vi "Untitled 2.vi"() -> ()   [LabVIEW 2020]
panel:
  in  "Numeric":i32
  out "XY Graph":cluster{"Y":dbl[], "Y":dbl[]}[](graph)
  in  "I0":dbl
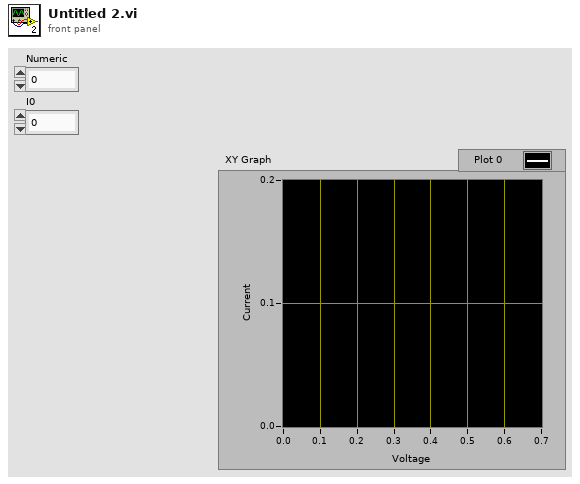
[diagram p1: front panel]
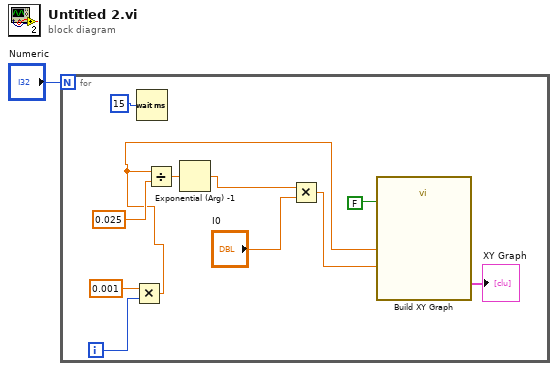
[diagram p0: block diagram]
diagram:
  n1 = for {
    N: "Numeric" -> [_]
    i -> [w5]
    n2 = Multiply(x=0.001, y=w5) -> (x*y=w4:dbl)
    n3 = Wait (ms)(milliseconds to wait=u32 15) -> ()  [unwired: 1 out]
    n4 = Divide(x=w4, y=0.025) -> (x/y=w11:dbl)
    n5 = Exponential (Arg) -1(1:w11) -> (0:w10:dbl)
    n6 = Multiply(x=w10, y="I0") -> (x*y=w7:dbl)
    n7 = call "Build XY Graph"("Reset"=FALSE, "Y Input"=w7, "X Input"=w4) -> ("XY Graph"=→"XY Graph":cluster{"X":dbl[], "Y":dbl[]}[])  [unwired: 7 in, 1 out]
  }
